vi "Delete Many Attributes Priv.vi"(0 "Tree Dictionary In":variant, 5 "Unique ID":string, 7 "Attribute Names":string[](array[string]), 11 "error in":errorcluster) -> (4 "Tree Dictionary Out":variant, 15 "error out":errorcluster)   [LabVIEW 2020, in "NI_VIAnCFGDataStructure.lvlib" / "Tree.lvclass"]
uses:
  <vilib>/addons/analyzer/VIAnCFGDataStructure/Tree Manager/Tree.lvclass
  <vilib>/addons/analyzer/VIAnCFGDataStructure/Tree Manager/Typedefs/Tree Cluster.ctl
  <vilib>/Utility/error.llb/Error Cluster From Error Code.vi
  <vilib>/ErrorRing/Error Ring.xnode
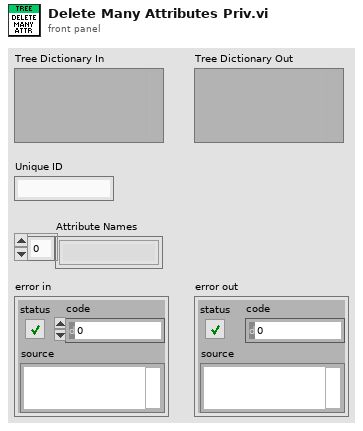
[diagram p1: front panel]
types:
  T1 = typedef "NI_VIAnCFGDataStructure.lvlib/Tree.lvclass/Tree Cluster.ctl" = cluster{"Unique ID":string, "Parent ID":string, "Child IDs":string[], "Name":string, "MetaData":string, "Data IDs":string[]}
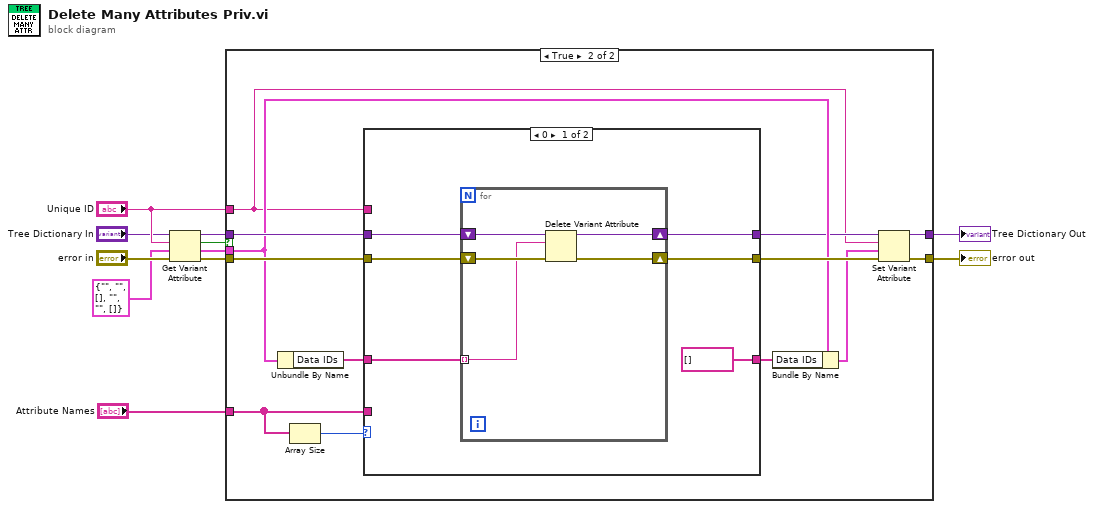
[diagram p0: block diagram]
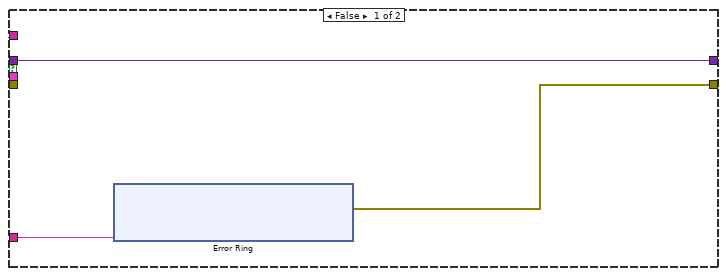
[diagram p2: hidden frame]
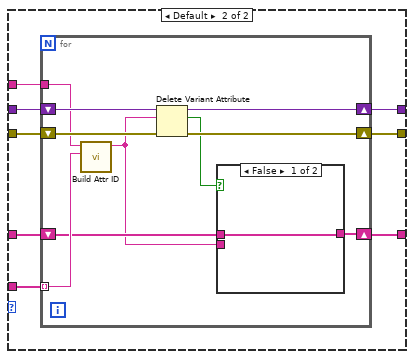
[diagram p3: hidden frame]
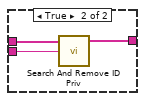
[diagram p4: hidden frame]
diagram:
  n1 = Get Variant Attribute(Variant="Tree Dictionary In", name="Unique ID", default value (empty Variant)=T1 {"Unique ID"="", "Parent ID"="", "Child IDs"=[], "Name"="", "MetaData"="", "Data IDs"=[]} ("Cluster of class private data"), error in="error in") -> (duplicate Variant=w8:variant, found=w9:bool, value=w10:T1, error out=w6:errorcluster)
  n2 = case shown="True" w9 {
    tunnel: [w13 w34] -> w4
    tunnel: [w14 w33] -> w5
    tunnel: w6 -> [_ w32]
    tunnel: w8 -> [w14 w27]
    tunnel: w10 -> [_ w26]
    tunnel: "Unique ID" -> [w12 w22]
    tunnel: "Attribute Names" -> [_ w29]
    frame False {
      n3 = xnode "Error Ring"("parameter 0"=w12) -> ("error out"=w13:errorcluster)
    }
    frame True {
      n4 = Unbundle By Name(w26) -> ("Data IDs"=w30:string[])
      n5 = Array Size(array=w29) -> (size(s)=w28:i32)
      n6 = case shown="0" w28 {
        tunnel: w32 -> [w40 w53]
        tunnel: [w39 w52] -> w31
        tunnel: w30 -> [w38 w47]
        tunnel: w29 -> [_ w51]
        tunnel: w27 -> [w37 w50]
        tunnel: [string[] [] ("Data IDs") w46] -> w25
        tunnel: [w35 w49] -> w23
        tunnel: w22 -> [_ w48]
        frame 0 {
          n7 = for {
            tunnel: w38 -> [w43] mode=indexing
            shift-right: [w44] -> w39
            shift-left: w40 -> [w45]
            shift-right: [w41] -> w35
            shift-left: w37 -> [w42]
            n8 = Delete Variant Attribute(4:w45, 6:w43, 7:w42) -> (0:w44:errorcluster, 3:w41:variant)  [unwired: 1 out]
          }
        }
        frame Default {
          n9 = for {
            shift-right: [w62] -> w52
            shift-left: w53 -> [w63]
            tunnel: w51 -> [w58] mode=indexing
            shift-right: [w60] -> w49
            shift-left: w50 -> [w61]
            tunnel: w48 -> [w59]
            shift-right: [w54] -> w46
            shift-left: w47 -> [w56]
            n10 = call <vilib>:"Build Attr ID.vi"("Attr Name"=w58, "Unique ID"=w59) -> ("Attr ID Out"=w55:string)  [unwired: 9 in]
            n11 = Delete Variant Attribute(4:w63, 6:w55, 7:w61) -> (0:w62:errorcluster, 2:w57:bool, 3:w60:variant)
            n12 = case shown="False" w57 {
              tunnel: w56 -> [w64 w67]
              tunnel: w55 -> [_ w66]
              tunnel: [w64 w65] -> w54
              frame False {
              }
              frame True {
                n13 = call <vilib>:"Search And Remove ID Priv.vi"("Remove String"=w66, "Strings In"=w67) -> ("Strings Out"=w65:string[])  [unwired: 3 in]
              }
            }
          }
        }
      }
      n14 = Bundle By Name(cluster=w26, "Data IDs"=w25) -> (w24:T1)
      n15 = Set Variant Attribute(Variant=w23, name=w22, value=w24, error in=w31) -> (Variant out=w33:variant, error out=w34:errorcluster)  [unwired: 1 out]
    }
  }
  "Tree Dictionary Out" <- w5
  "error out" <- w4
